vi "RLC.vi"() -> ()   [LabVIEW 2011]
uses:
  <vilib>/Analysis/NI_AALBase.lvlib
panel:
  out "step":timestamp
  out "total time":timestamp
  out "start":timestamp format="%<%H:%M:%S\n%x>T"
  out "end":timestamp
  out "time stamp 2":timestamp[](array[timestamp])
  out "t":dbl[](array[numeric])
  out "I":dbl[](array[numeric])
  out "V":dbl[](array[numeric])
  out "R":dbl[](array[numeric])
  out "C":dbl[](array[numeric])
  out "MEASURE I [A]":dbl
  out "MEASURE V [V]":dbl
  out "MEASURE R [Ohm ]":dbl
  in  "Tab Control":T1(tab)
  in  "Sample name":string
  in  "File name_CDH":string
  in  "Nota 01":string
  in  "Nota 2":string
  in  "Nota 3":string
  in  "new file":bool
  out "path":path
  out "Waveform Chart":dynamicdata(graph)
  in  "read RLC":bool
  in  "Close RLC 2":bool
  in  "Ligar RLC":bool
  out "RLC300 - digimess":string
  in  "New Button":bool
  in  "Tab Control 2":enum32{"C x R", "C x I", "C x V", "Filtro"}(tab)
  out "XY Graph":cluster{dbl[], dbl[]}(graph)
  out "XY Graph 2":cluster{dbl[], dbl[]}(graph)
  out "XY Graph 3":cluster{dbl[], dbl[]}(graph)
  out "filtro":dbl[][](graph)
  in  "Filter Rank":i32(slide)=7 scale=0.0..100.0
  in  "Refresh Button":bool
  in  "New Button 2":bool
  out "MEASURE C [F ] 2":dbl
  in  "stop":bool
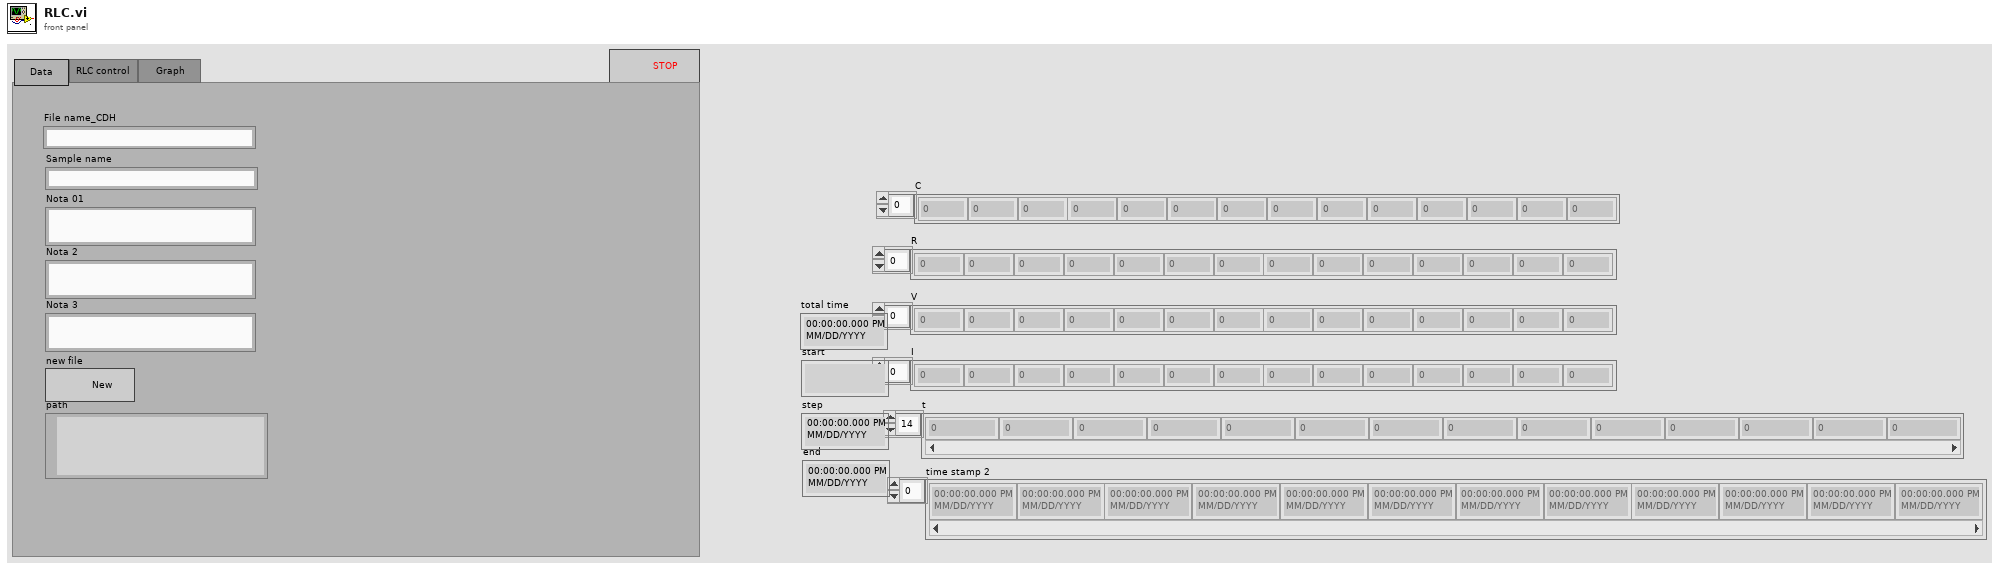
[diagram p1: front panel]
types:
  T1 = enum32{"Data       ", "RLC control ", "Graph        "}
  T2 = enum16{"open", "replace", "create", "open or create", "replace or create", "replace or create with confirmation"}
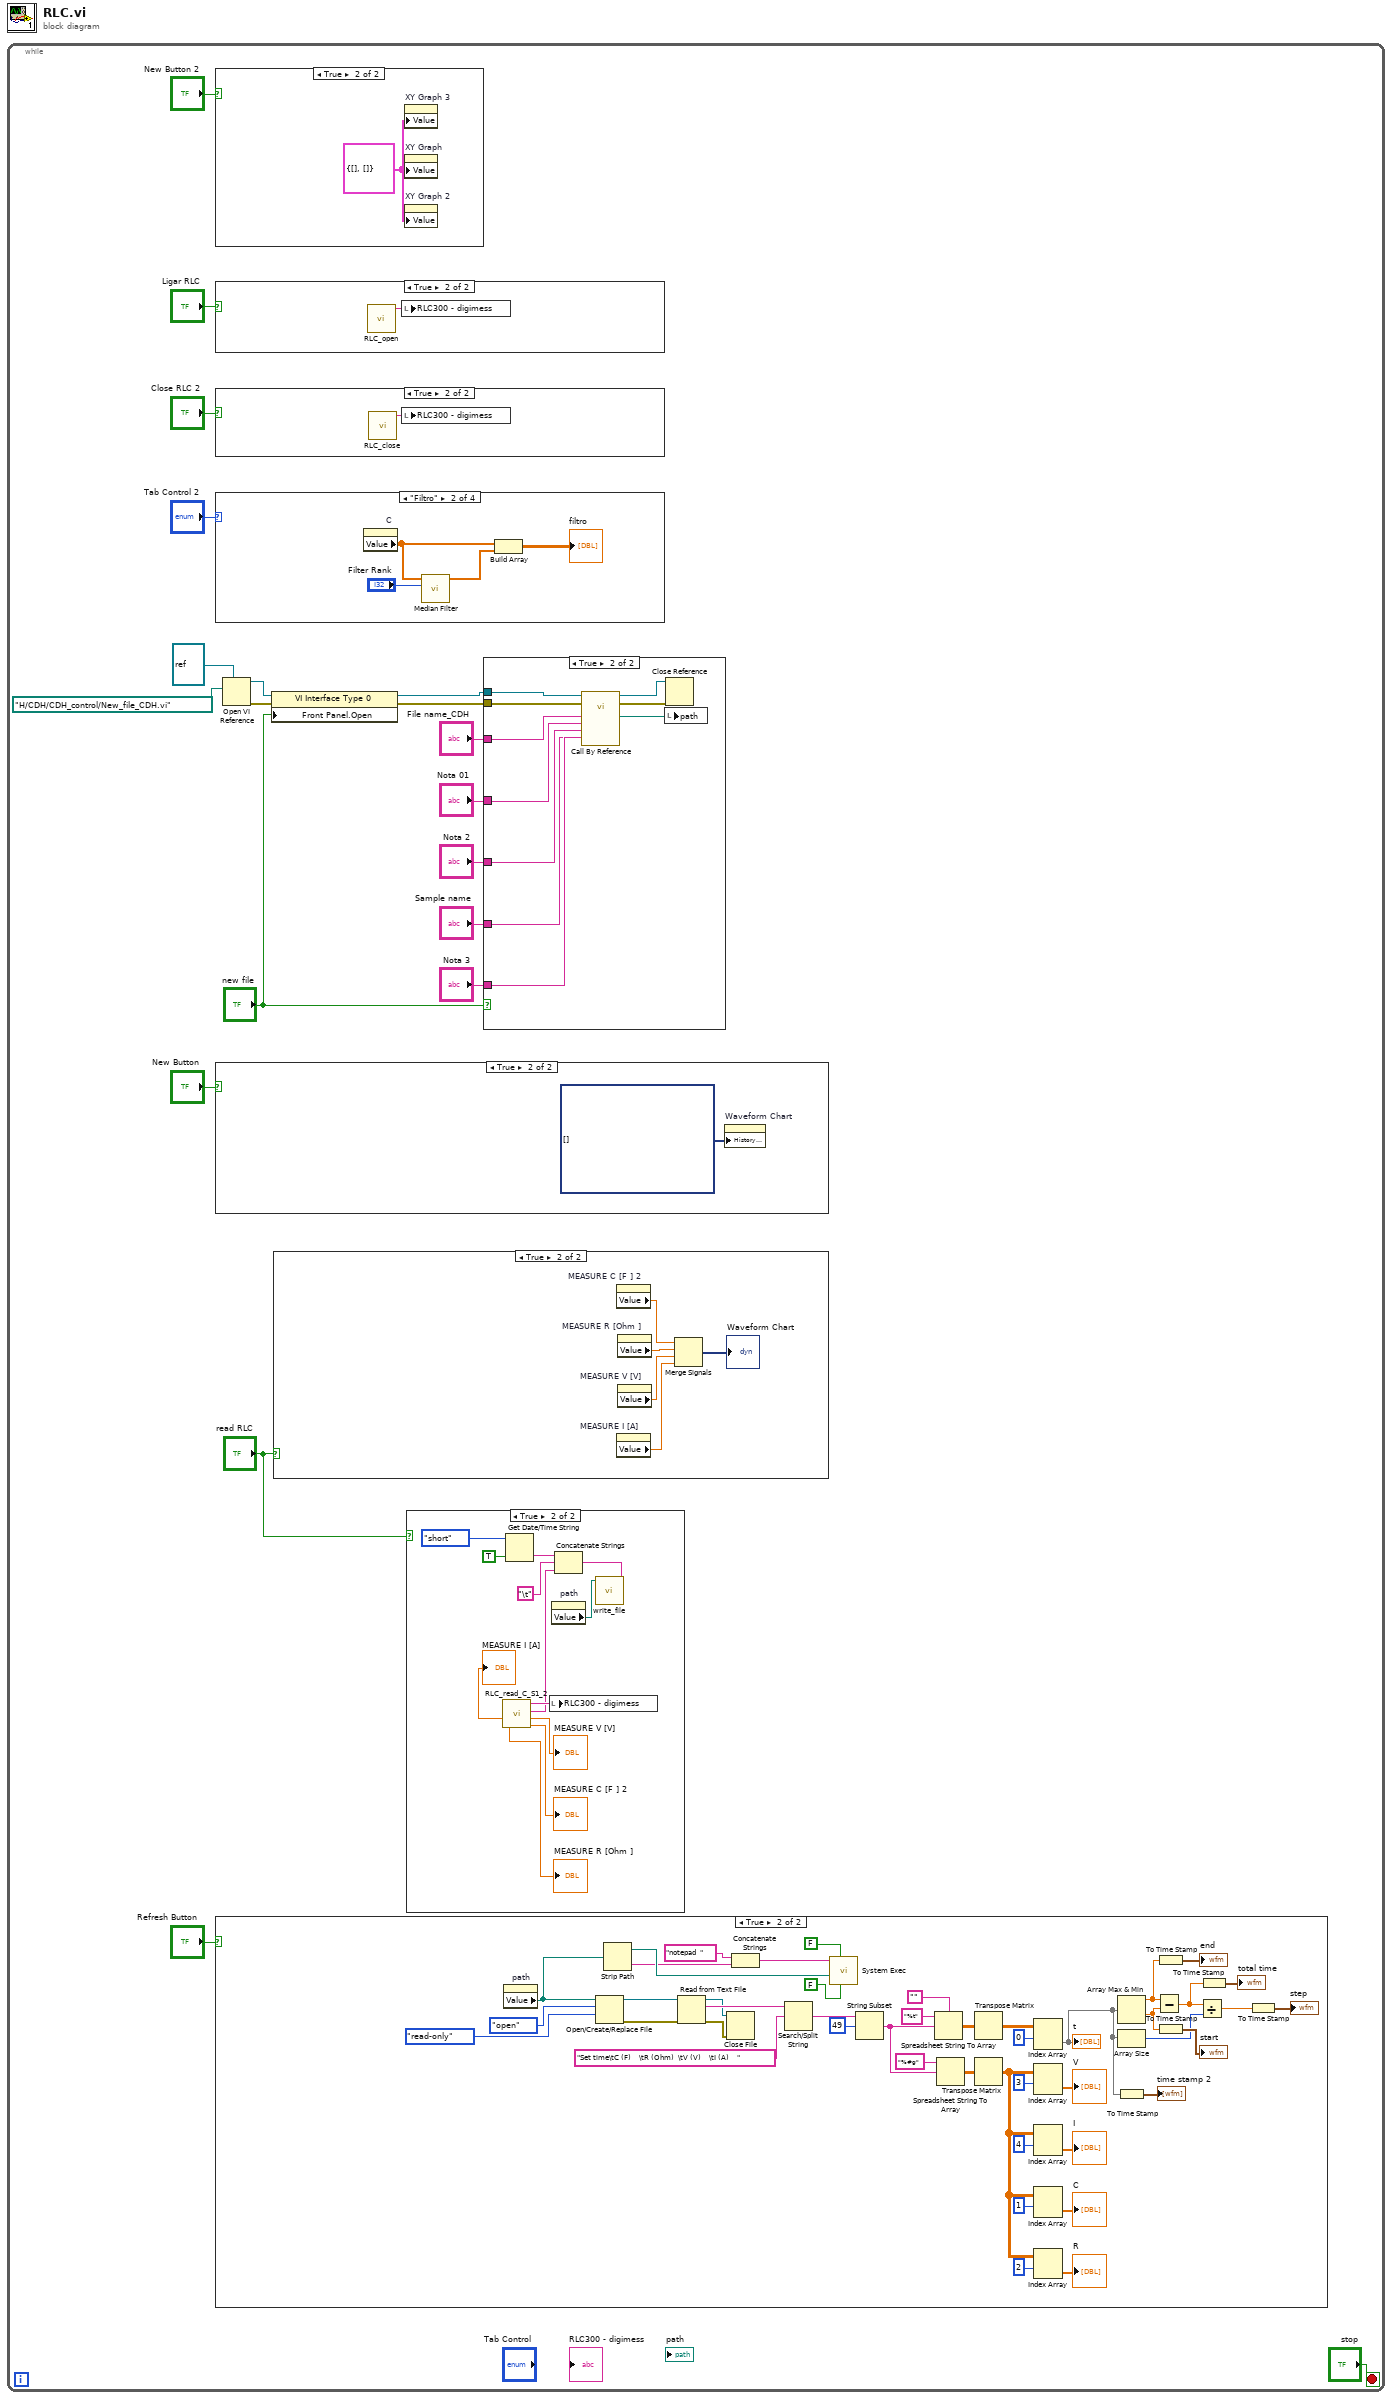
[diagram p0: block diagram]
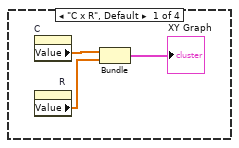
[diagram p2: hidden frame]
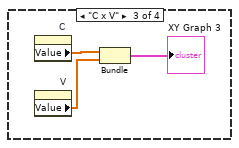
[diagram p3: hidden frame]
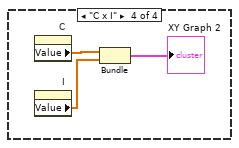
[diagram p4: hidden frame]
diagram:
  n1 = while {
    stop <- "stop" stop-if-true
    n2 = case shown="True" "New Button 2" {
      frame False {
      }
      frame True {
        w34 = cluster{dbl[], dbl[]} {[], []} ("XY Graph")
        n3 = property on="XY Graph 3" class="XYGraph (strict)"("Value"=w34) -> ()  [unwired: 2 in, 2 out]
        n4 = property on="XY Graph" class="XYGraph (strict)"("Value"=w34) -> ()  [unwired: 2 in, 2 out]
        n5 = property on="XY Graph 2" class="XYGraph (strict)"("Value"=w34) -> ()  [unwired: 2 in, 2 out]
      }
    }
    n6 = case shown="True" "Ligar RLC" {
      frame False {
      }
      frame True {
        n7 = call "RLC_open.vi"() -> ("String 2"=w97:string)  [unwired: 10 in, 1 out]
        n8 = local write "RLC300 - digimess"(w97) -> ()
      }
    }
    n9 = case shown="True" "Close RLC 2" {
      frame False {
      }
      frame True {
        n10 = call "RLC_close.vi"() -> ("String"=w81:string)  [unwired: 11 in]
        n11 = local write "RLC300 - digimess"(w81) -> ()
      }
    }
    n12 = case shown="\"Filtro\"" "Tab Control 2" {
      frame "C x R", Default {
        n13 = property on="C" class="Arr (strict)"() -> ("Value"=w22:dbl[])  [unwired: 2 in, 2 out]
        n14 = property on="R" class="Arr (strict)"() -> ("Value"=w21:dbl[])  [unwired: 2 in, 2 out]
        n15 = Bundle("Value"=w22, "Value"=w21) -> (→"XY Graph":cluster{"Value":dbl[], "Value":dbl[]})  [unwired: 1 in]
      }
      frame "Filtro" {
        n16 = property on="C" class="Arr (strict)"() -> ("Value"=w25:dbl[])  [unwired: 2 in, 2 out]
        n17 = call <vilib>:"Median Filter.vi"("left rank"="Filter Rank", "X"=w25) -> ("Filtered X"=w26:dbl[])  [unwired: 8 in, 1 out]
        n18 = Build Array(w25, w26) -> (→"filtro":dbl[][])
      }
      frame "C x V" {
        n19 = property on="C" class="Arr (strict)"() -> ("Value"=w30:dbl[])  [unwired: 2 in, 2 out]
        n20 = property on="V" class="Arr (strict)"() -> ("Value"=w29:dbl[])  [unwired: 2 in, 2 out]
        n21 = Bundle("Value"=w30, "Value"=w29) -> (→"XY Graph 3":cluster{"Value":dbl[], "Value":dbl[]})  [unwired: 1 in]
      }
      frame "C x I" {
        n22 = property on="C" class="Arr (strict)"() -> ("Value"=w33:dbl[])  [unwired: 2 in, 2 out]
        n23 = property on="I" class="Arr (strict)"() -> ("Value"=w32:dbl[])  [unwired: 2 in, 2 out]
        n24 = Bundle("Value"=w33, "Value"=w32) -> (→"XY Graph 2":cluster{"Value":dbl[], "Value":dbl[]})  [unwired: 1 in]
      }
    }
    n25 = case shown="True" "New Button" {
      frame False {
      }
      frame True {
        n26 = property on="Waveform Chart" class="WFChart (strict)"("History Data"=dynamicdata[] []) -> ()  [unwired: 2 in, 2 out]
      }
    }
    n27 = case shown="True" "Refresh Button" {
      frame False {
      }
      frame True {
        n28 = property on="path" class="Path"() -> ("Value"=w71:path)  [unwired: 2 in, 2 out]
        n29 = Open/Create/Replace File(file path (use dialog)=w71, operation (0:open)=T2."open", access (0:read/write)=enum16{"read/write", "read-only", "write-only"}."read-only") -> (refnum out=w76:refnum<file>, error out=w77:errorcluster)  [unwired: 3 in, 1 out]
        n30 = Strip Path(path=w71) -> (stripped path=w72:path, name=w70:string)
        n31 = Read from Text File(file (use dialog)=w76, error in=w77) -> (refnum out=w65:refnum<file>, text=w69:string, error out=w66:errorcluster)  [unwired: 2 in, 1 out]
        n32 = Close File(refnum=w65, error in=w66) -> ()  [unwired: 2 out]
        n33 = Concatenate Strings("notepad  ", w70) -> (w74:string)
        n34 = Search/Split String(string=w69, search string/char (-)="Set time\tC (F)    \tR (Ohm)  \tV (V)    \tI (A)    ") -> (match + rest of string=w64:string)  [unwired: 1 in, 2 out]
        n35 = call <vilib>:"System Exec.vi"("run minimized? (F)"=FALSE ("Boolean"), "wait until completion? (T)"=FALSE, "working directory"=w72, "command line"=w74) -> ()  [unwired: 4 in, 4 out]
        n36 = String Subset(string=w64, offset (0)=49) -> (substring=w35:string)  [unwired: 1 in]
        n37 = Spreadsheet String To Array(delimiter (Tab)="", format string="%t", spreadsheet string=w35) -> (array=w48:dbl[][])  [unwired: 1 in]
        n38 = Spreadsheet String To Array(format string="%#g", spreadsheet string=w35) -> (array=w54:dbl[][])  [unwired: 2 in]
        n39 = Transpose Matrix(1:w48) -> (0:w47:dbl[][])
        n40 = Transpose Matrix(1:w54) -> (0:w55:dbl[][])
        n41 = Index Array(array=w47, index (row)=0 ("index (row) 2")) -> (element=w37:dbl[])  [unwired: 1 in]
        "t" <- w37
        n42 = Index Array(array=w55, index (row)=3 ("index (row) 4")) -> (element=→"V":dbl[])  [unwired: 1 in]
        n43 = Index Array(array=w55, index (row)=4 ("index (row) 5")) -> (element=→"I":dbl[])  [unwired: 1 in]
        n44 = Index Array(array=w55, index (row)=1 ("index (row) 2")) -> (element=→"C":dbl[])  [unwired: 1 in]
        n45 = Index Array(array=w55, index (row)=2 ("index (row) 3")) -> (element=→"R":dbl[])  [unwired: 1 in]
        n46 = Array Max & Min(array=w37) -> (max value=w44:dbl, min value=w43:dbl)  [unwired: 2 out]
        n47 = Array Size(array=w37) -> (size(s)=w40:i32)
        n48 = To Time Stamp(1:w37) -> (0:→"time stamp 2":timestamp[])
        n49 = Subtract(x=w44, y=w43) -> (x-y=w41:dbl)
        n50 = To Time Stamp(1:w44) -> (0:→"end":timestamp)
        n51 = To Time Stamp(1:w43) -> (0:→"start":timestamp)
        n52 = Divide(x=w41, y=w40) -> (x/y=w39:dbl)
        n53 = To Time Stamp(1:w41) -> (0:→"total time":timestamp)
        n54 = To Time Stamp(1:w39) -> (0:→"step":timestamp)
      }
    }
    n55 = Open VI Reference(type specifier VI Refnum (for type only)=refnum<vi> refnum ("application reference (local)"), vi path=path "H:/CDH/CDH_control/New_file_CDH.vi" ("vi path 2")) -> (vi reference=w17:refnum<vi>, error out=w16:errorcluster)  [unwired: 4 in]
    n56 = property class="VI Interface Type 0"(reference=w17, error in=w16, "Front Panel.Open"="new file") -> (reference out=w13:refnum<vi>, error out=w14:errorcluster)
    n57 = case shown="True" "read RLC" {
      frame False {
      }
      frame True {
        n58 = property on="MEASURE C [F ] 2" class="DigNum (strict)"() -> ("Value"=w85:dbl)  [unwired: 2 in, 2 out]
        n59 = property on="MEASURE I [A]" class="DigNum (strict)"() -> ("Value"=w82:dbl)  [unwired: 2 in, 2 out]
        n60 = property on="MEASURE R [Ohm ]" class="DigNum (strict)"() -> ("Value"=w84:dbl)  [unwired: 2 in, 2 out]
        n61 = property on="MEASURE V [V]" class="DigNum (strict)"() -> ("Value"=w83:dbl)  [unwired: 2 in, 2 out]
        n62 = Merge Signals(w85, w84, w83, w82) -> (→"Waveform Chart":dynamicdata)
      }
    }
    n63 = case shown="True" "read RLC" {
      frame False {
      }
      frame True {
        n64 = call "RLC_read_C_S1_2.vi"() -> ("MEASURE C [F ]"=→"MEASURE C [F ] 2":dbl, "MEASURE V [V]"=→"MEASURE V [V]":dbl, "concatenated string"=w102:string, "READ RLC300 - digimess"=w103:string, "MEASURE R [Ohm ]"=→"MEASURE R [Ohm ]":dbl, "MEASURE I [A]"=→"MEASURE I [A]":dbl)  [unwired: 2 in]
        n65 = Get Date/Time String(date format (0)=enum16{"short", "long", "abbreviated"}."short", want seconds? (F)=TRUE) -> (time string=w105:string)  [unwired: 1 in, 1 out]
        n66 = local write "RLC300 - digimess"(w103) -> ()
        n67 = property on="path" class="Path"() -> ("Value"=w104:path)  [unwired: 2 in, 2 out]
        n68 = Concatenate Strings(w105, "\t", w102) -> (w106:string)
        n69 = call "write_file.vi"("dados_ CDH"=w106, "file path (use dialog)"=w104) -> ()  [unwired: 10 in]
      }
    }
    n70 = case shown="True" "new file" {
      tunnel: w13 -> [_ w96]
      tunnel: w14 -> [_ w95]
      tunnel: "File name_CDH" -> [_ w92]
      tunnel: "Nota 2" -> [_ w91]
      tunnel: "Nota 01" -> [_ w90]
      tunnel: "Nota 3" -> [_ w89]
      tunnel: "Sample name" -> [_ w88]
      frame False {
      }
      frame True {
        n71 = call-by-ref "?"(reference=w96, error in=w95, "Sample name"=w88, "Nota 3"=w89, "Nota 2"=w91, "Nota 01"=w90, "File name"=w92) -> (reference out=w93:refnum<vi>, error out=w94:errorcluster, "path"=w87:path)  [unwired: 6 in]
        n72 = local write "path"(w87) -> ()
        n73 = Close Reference(reference=w93, error in (no error)=w94) -> ()  [unwired: 1 out]
      }
    }
  }
